vi "Add Copyright.vi"() -> ()   [LabVIEW 2016]
uses:
  SLL Tools/Copyright/_Typedefs/Select File Type.ctl
  <vilib>/Utility/error.llb/DialogType.ctl
  SLL Queued State Machine/Queue Driver/Create Queue.vi
  SLL Queued State Machine/Queue Driver/Enqueue an Item to Queue.vi
  SLL Queued State Machine/Queue Driver/Dequeue Queue.vi
  SLL Queued State Machine/Queue Driver/Enqueue N Items.vi
  SLL Queued State Machine/Queue Driver/Flush Queue.vi
  SLL Queued State Machine/Queue Driver/Release Queue.vi
  SLL Queued State Machine/SLL QSM.lvlib
  SLL Tools/Copyright/SLL Add Copyright.lvlib
panel:
  in  "Type":T1={"vi"=TRUE, "ctl"=TRUE, "lvlib"=TRUE, "lvclass"=TRUE, "lvproj"=TRUE} caption="Select File Type to Add Copyright"
  in  "Copyright Text":string="© Company Name"
  in  "Source Code Directory":path
  out "Status":string
  in  "Run":bool
  # "Add Copyright"
  # "Adds/updates copyright text to LabVIEW Files (VIs, Controls, Libraries, Classes and Projects)"
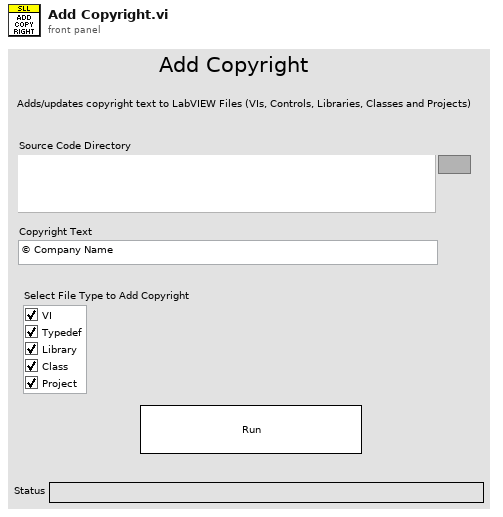
[diagram p1: front panel]
types:
  T1 = typedef "SLL Add Copyright.lvlib/Select File Type.ctl" = cluster{"vi":bool, "ctl":bool, "lvlib":bool, "lvclass":bool, "lvproj":bool}
  T2 = typedef "DialogType.ctl" = u16
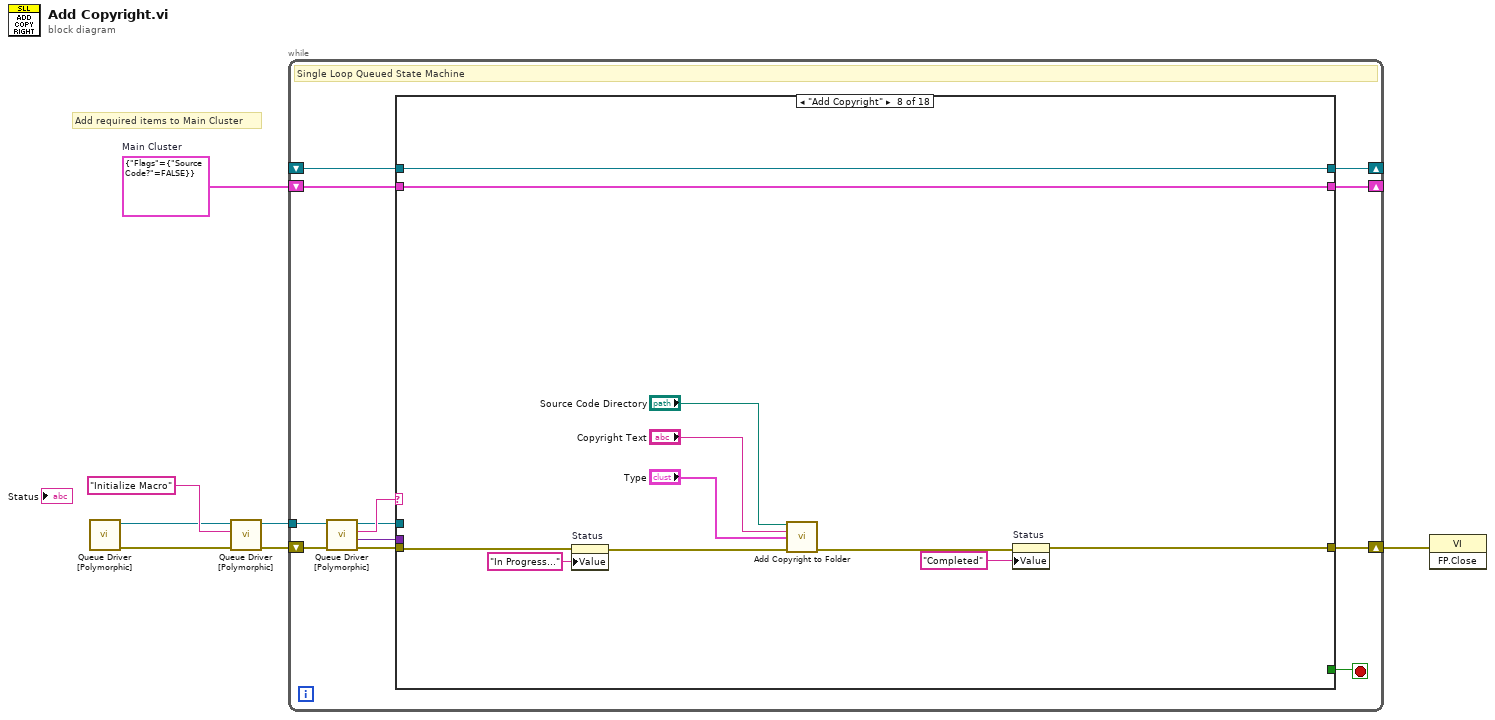
[diagram p0: block diagram]
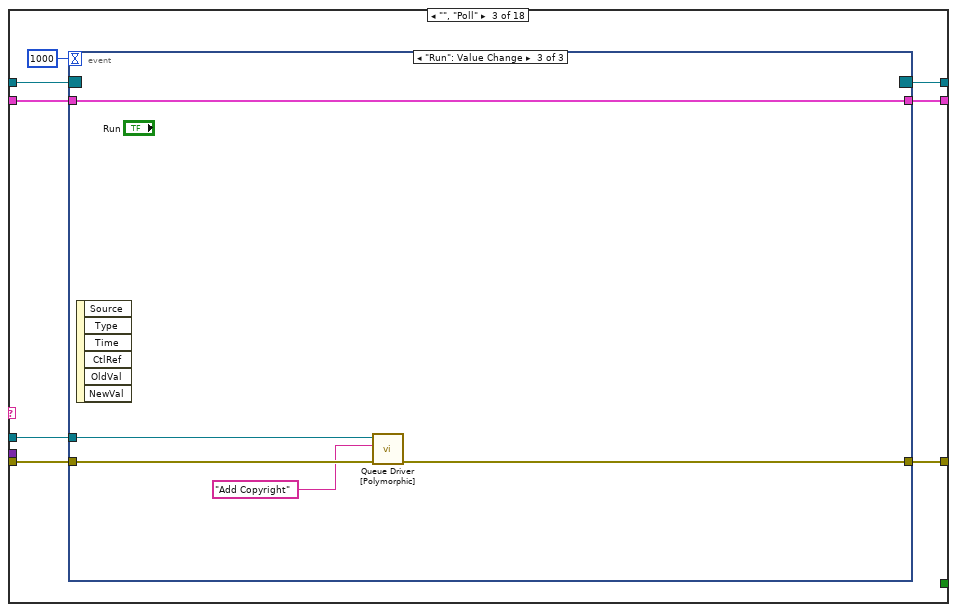
[diagram p4: hidden frame]
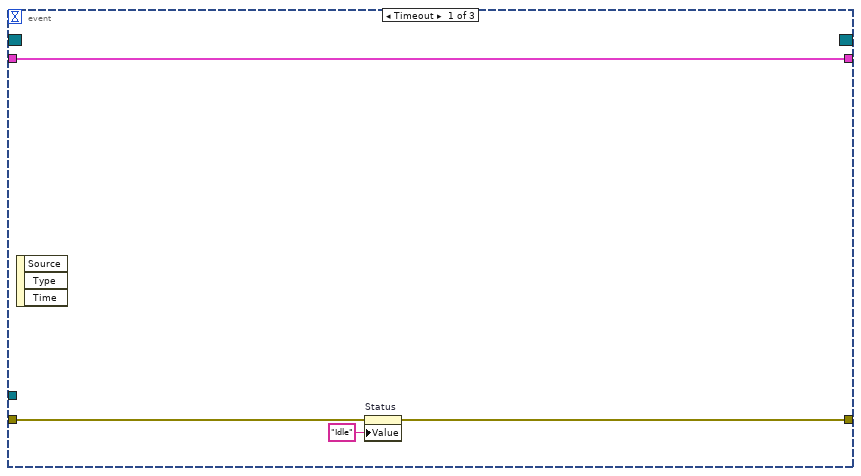
[diagram p5: hidden frame]
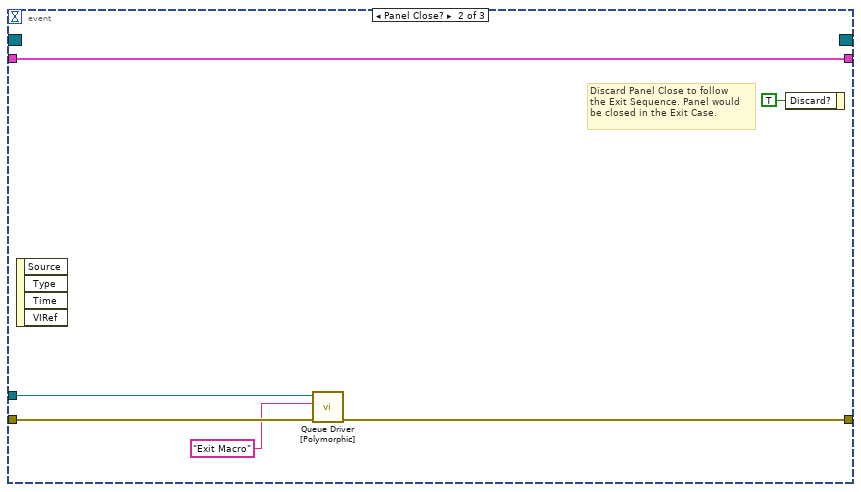
[diagram p6: hidden frame]
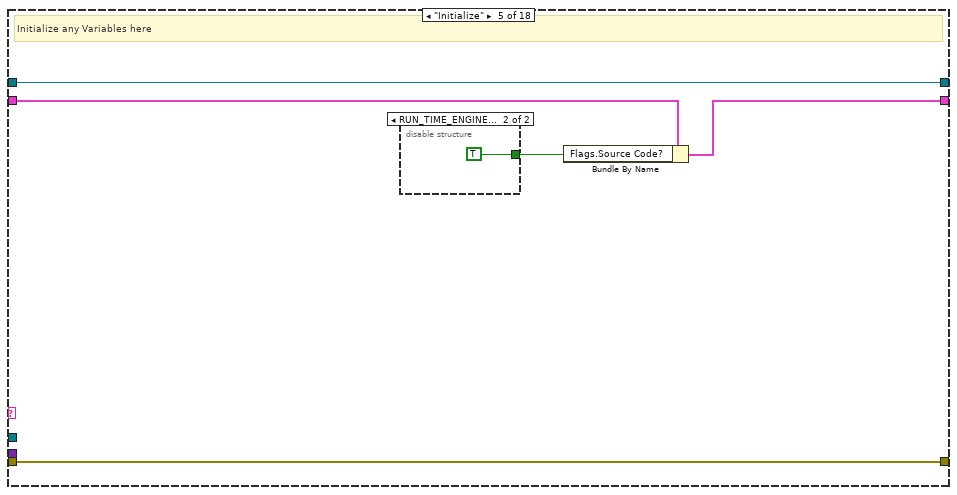
[diagram p8: hidden frame]
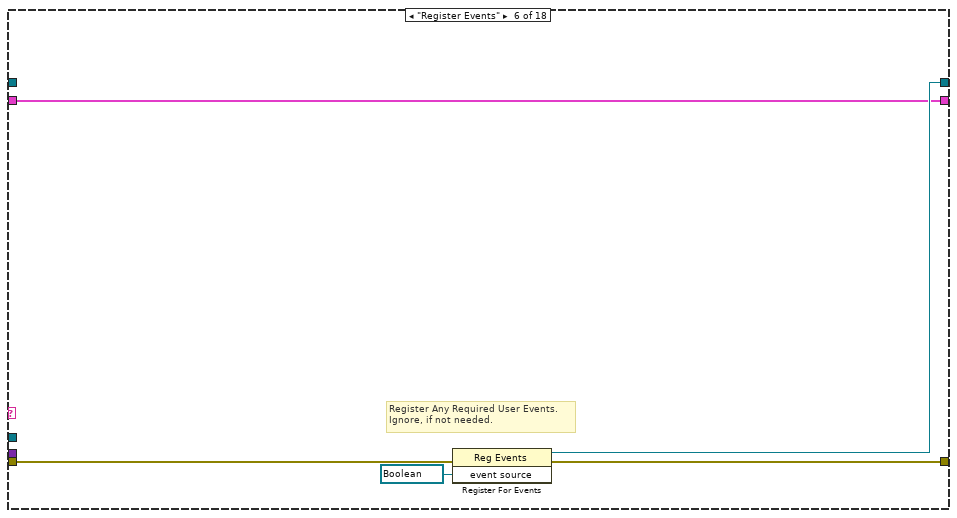
[diagram p10: hidden frame]
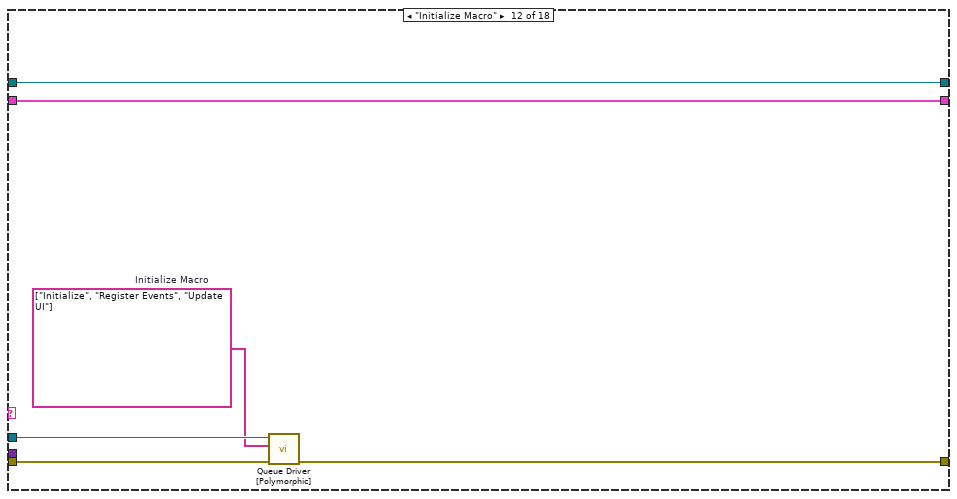
[diagram p15: hidden frame]
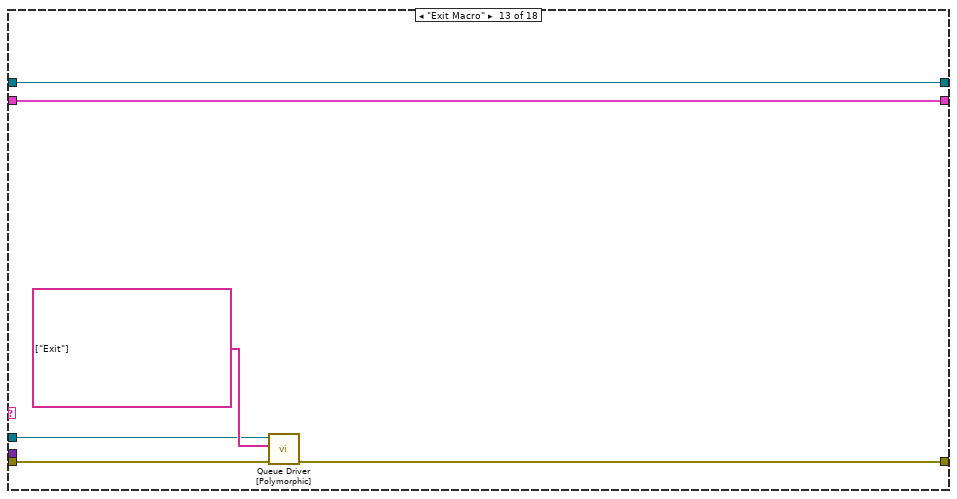
[diagram p16: hidden frame]
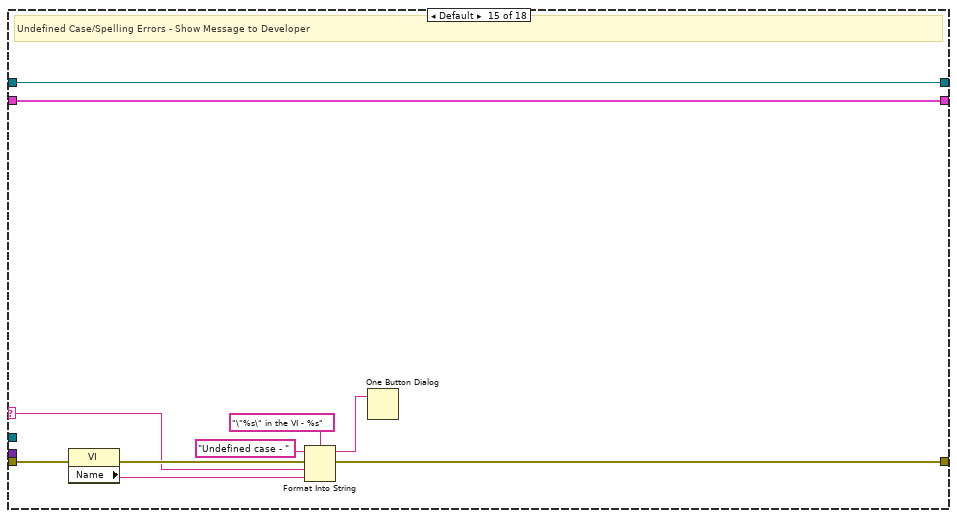
[diagram p18: hidden frame]
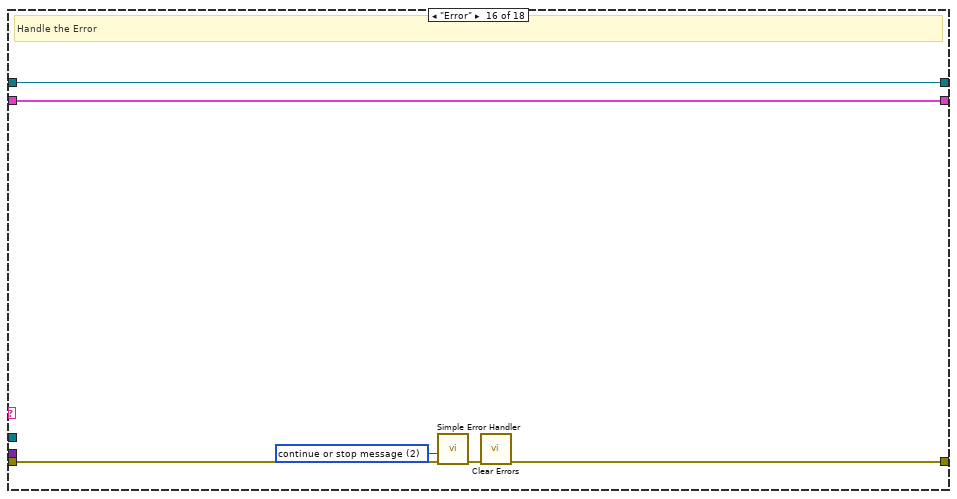
[diagram p19: hidden frame]
diagram:
  w5 = cluster{"Flags":cluster{"Source Code?":bool}} {"Flags"={"Source Code?"=FALSE}}  # Main Cluster
  # "Add required items to Main Cluster"
  n1 = call-poly "Queue Driver [Polymorphic].vi"() -> ("Error Out"=w7:errorcluster, "Queue Ref"=w3:refnum<queue>)  [unwired: 10 in]
  n2 = call-poly "Queue Driver [Polymorphic].vi"("Error In"=w7, "Item to Add"="Initialize Macro", "Queue Ref In"=w3) -> ("Error Out"=w6:errorcluster, "Queue Ref Out"=w2:refnum<queue>)  [unwired: 7 in]
  n3 = while "SLL Queued State Machine" {
    shift-right: [w17] -> w1
    shift-left: w6 -> [w19]
    shift-right: [w15] -> _
    shift-left: _ -> [w14]
    shift-right: [w13] -> _
    shift-left: w5 -> [w12]
    tunnel: w2 -> [w10]
    stop <- w16 stop-if-true
    # "Single Loop Queued State Machine"
    n4 = call-poly "Queue Driver [Polymorphic].vi"("Error In"=w19, "Queue Ref In"=w10) -> ("Error Out"=w18:errorcluster, "Data"=w8:variant, "Dequeue"=w11:string, "Queue Ref Out"=w9:refnum<queue>)  [unwired: 6 in]
    n5 = case "QSM Case Structure" shown="\"Add Copyright\"" w11 {
      selector: w11 -> [_ _ _ _ _ _ _ _ _ _ _ _ _ _ w101 _ _ _]
      tunnel: w18 -> [w22 w25 w31 w51 w56 w62 w65 w73 w79 w82 w85 w89 w95 w100 w104 w116 w119 w132]
      tunnel: [w22 w25 w32 w51 w56 w61 w65 w71 w79 w82 w85 w88 w94 w100 w107 w114 w119 w128] -> w17
      tunnel: [_ _ _ _ _ _ _ _ _ _ _ _ _ _ _ _ _ TRUE] -> w16
      tunnel: [w21 w24 w30 w50 w55 w60 w64 w76 w78 w81 w84 w91 w97 w99 w110 w113 w118 w131] -> w15
      tunnel: w14 -> [w21 w24 w29 w50 w55 _ w64 w76 w78 w81 w84 w91 w97 w99 w110 w113 w118 w131]
      tunnel: [w20 w23 w27 w49 w52 w59 w63 w75 w77 w80 w83 w90 w96 w98 w109 w112 w117 w130] -> w13
      tunnel: w12 -> [w20 w23 w28 w49 w53 w59 w63 w75 w77 w80 w83 w90 w96 w98 w109 w112 w117 w130]
      tunnel: w9 -> [_ _ w26 _ _ _ _ _ _ _ _ w87 w92 _ _ _ _ w121]
      tunnel: w8 -> [_ _ _ _ _ _ _ _ _ _ _ _ _ _ _ _ _ _]
      frame "/--------------- Read Me -----------------/" {
        # "General Purpose Queue Based State Machine for Any Use Case (main application, module, pop up message etc)\n\nAdvantages:\n1. No Need to Pass Queue References between Queue Driver VIs.\n2. This template can be safely used in multiple parallel running modules without any issues.\n3. This template can also be safely used even in cases where the VI is configured to be a Clone, where multiple \ninstances of the VI could be executing concurrently.\n\nHow to Use:\n1. Add necessary items to the Main Cluster.\n2. Use the Polymorphic Queue Driver for doing any queue operations. There is no need to pass the queue driver\nreference, as the Queue Driver automatically infers the reference based on the VI instance from which it is called.\n3. Add any required user events in the \"Register Events\" case. Ignore if not needed.\n4. Use \"Sequences\" section for defining any list of state calls, which could be used in multiple places. \nEg: Initialize Sequence, might be needed if we need to any reinitialization."
      }
      frame "/------------------ Poll -------------------/" {
      }
      frame "", "Poll" {
        n6 = event shown="[2] \"Run\": Value Change" {
          selector: w29 -> [_ _ _]
          dyn-events: [_ _ _] -> w30
          timeout: 1000 -> [_ _ _]
          tunnel: [w34 w42 w47] -> w32
          tunnel: w31 -> [w35 w43 w48]
          tunnel: w28 -> [w37 w41 w46]
          tunnel: [w37 w41 w46] -> w27
          tunnel: w26 -> [_ w38 w44]
          event Timeout {
            n7 = event-data() -> ()  [unwired: 1 in, 3 out]
            n8 = property on="Status" class="Str"(error in=w35, "Value"="Idle" ("Status")) -> (error out=w34:errorcluster)  [unwired: 1 in, 1 out]
          }
          event Panel Close? {
            # "Discard Panel Close to follow\nthe Exit Sequence. Panel would\nbe closed in the Exit Case."
            n9 = event-data() -> ()  [unwired: 1 in, 4 out]
            n10 = call-poly "Queue Driver [Polymorphic].vi"("Error In"=w43, "Item to Add"="Exit Macro" ("Enqueue"), "Queue Ref In"=w38) -> ("Error Out"=w42:errorcluster)  [unwired: 7 in, 1 out]
            n11 = event-data("Discard?"=TRUE) -> ()  [unwired: 1 in, 1 out]
          }
          event "Run": Value Change {
            n12 = event-data() -> ()  [unwired: 1 in, 6 out]
            n13 = call-poly "Queue Driver [Polymorphic].vi"("Error In"=w48, "Item to Add"="Add Copyright" ("Enqueue"), "Queue Ref In"=w44) -> ("Error Out"=w47:errorcluster)  [unwired: 7 in, 1 out]
          }
        }
      }
      frame "/--------------- Initialize -----------------/" {
      }
      frame "Initialize" {
        # "Initialize any Variables here"
        n14 = disable-structure shown="RUN_TIME_ENGINE==False" {
          disable-tunnel: [_ TRUE] -> w54
          frame condition #0 {
          }
          frame condition #1 (active) {
          }
        }
        n15 = Bundle By Name(cluster=w53, "Flags.Source Code?"=w54) -> (w52:cluster{"Flags":cluster{"Source Code?":bool}})
      }
      frame "Register Events" {
        # "Register Any Required User Events. \nIgnore, if not needed."
        n16 = register-events(error in=w62, refnum<vi> refnum ("event source")) -> (reference out=w60:refnum<event-registration>, error out=w61:errorcluster)  [unwired: 1 in]
      }
      frame "/---------- Custom Case Splitter ----------/" {
      }
      frame "Add Copyright" {
        n17 = property on="Status" class="Str"(error in=w73, "Value"="In Progress..." ("Status")) -> (error out=w74:errorcluster)  [unwired: 1 in, 1 out]
        n18 = call "Add Copyright to Folder.vi"("Source Code Directory"="Source Code Directory", "Copyright Text"="Copyright Text", "Type"="Type", "error in (no error)"=w74) -> ("error out"=w69:errorcluster)  [unwired: 11 in]
        n19 = property on="Status" class="Str"(error in=w69, "Value"="Completed" ("Status")) -> (error out=w71:errorcluster)  [unwired: 1 in, 1 out]
      }
      frame "/-------------- User Interface --------------/" {
        # "Duplicate this case to create additional case splitters for readability"
      }
      frame "Update UI" {
        # "Update Front Panel Controls in this Case"
      }
      frame "/----------------- Macros -----------------/" {
      }
      frame "Initialize Macro" {
        w86 = string[] ["Initialize", "Register Events", "Update UI"]  # Initialize Macro
        n20 = call-poly "Queue Driver [Polymorphic].vi"("Error In"=w89, "Enqueue N"=w86, "Queue Ref In"=w87) -> ("Error Out"=w88:errorcluster)  [unwired: 7 in, 1 out]
      }
      frame "Exit Macro" {
        n21 = call-poly "Queue Driver [Polymorphic].vi"("Error In"=w95, "Enqueue N"=string[] ["Exit"], "Queue Ref In"=w92) -> ("Error Out"=w94:errorcluster)  [unwired: 7 in, 1 out]
      }
      frame "/-------------- Error Handler--------------/" {
      }
      frame Default {
        # "Undefined Case/Spelling Errors - Show Message to Developer"
        n22 = property class="VI"(error in=w104) -> (error out=w103:errorcluster, "Name"=w102:string)  [unwired: 1 in, 1 out]
        n23 = Format Into String(format string="\"%s\" in the VI - %s" ("message"), initial string="Undefined case - ", error in=w103, w101, w102) -> (resulting string=w105:string, error out=w107:errorcluster)
        n24 = One Button Dialog(message=w105) -> ()  [unwired: 1 in, 1 out]
      }
      frame "Error" {
        w111 = T2 2 items=["no dialog", "OK message", "continue or stop message", "OK message + warnings", "continue/stop + warnings"] ("type of dialog (OK msg:1)")
        # "Handle the Error"
        n25 = call <vilib>:"Simple Error Handler.vi"("type of dialog (OK msg:1)"=w111, "error in (no error)"=w116) -> ("error out"=w115:errorcluster)  [unwired: 3 in, 4 out]
        n26 = call <vilib>:"Clear Errors.vi"("error in (no error)"=w115) -> ("error out"=w114:errorcluster)  [unwired: 5 in, 1 out]
      }
      frame "/------------------- Exit --------------------/" {
      }
      frame "Exit" {
        n27 = call-poly "Queue Driver [Polymorphic].vi"("Error In"=w132, "Queue Ref In"=w121) -> ("Error Out"=w133:errorcluster, "Queue Ref Out"=w120:refnum<queue>)  [unwired: 7 in, 1 out]
        n28 = Unbundle By Name(w130) -> ("Flags.Source Code?"=w123:bool)
        n29 = call-poly "Queue Driver [Polymorphic].vi"("Error In"=w133, "Queue Ref In"=w120) -> ("Error Out"=w129:errorcluster)  [unwired: 9 in]
        n30 = Call Chain() -> (call chain=w127:string[])
        n31 = Array Size(array=w127) -> (size(s)=w126:i32)
        n32 = Equal?(x=w126, y=1) -> (x = y?=w124:bool)
        n33 = And(x=w123, y=w124) -> (x .and. y?=w122:bool)
        n34 = case "Skip Panel Close when in Source\nCode and is the top most caller" shown="True" w122 {
          tunnel: w129 -> [w136 w138]
          tunnel: [w137 w138] -> w128
          frame False {
            # "Close Panel"
            n35 = invoke class="VI" method="FP.Close"() -> (error out=w135:errorcluster)  [unwired: 3 in, 2 out]
            n36 = Merge Errors(w136, w135) -> (w137:errorcluster)
          }
          frame True {
            # "Do Not Close Panel"
          }
        }
      }
    }
  }
  n37 = invoke class="VI" method="FP.Close"(error in=w1) -> ()  [unwired: 2 in, 3 out]
